vi "Delete.vi"(0 "video in":refnum<class "MSC Video.lvclass">, 5 "error in (no error)":errorcluster) -> (19 "error out":errorcluster)   [LabVIEW 2014, in "MSC Video.lvclass"]
doc: "Closes the video reference and frees occupied memory.\nUse this function for each initialized video to prevent memory leaks."
uses:
  MSC Video.lvclass
  MSC Video.lvclass/MSC Video.ctl
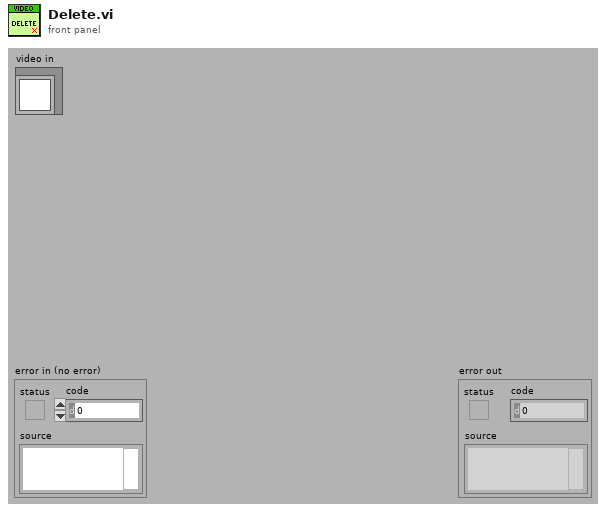
[diagram p1: front panel]
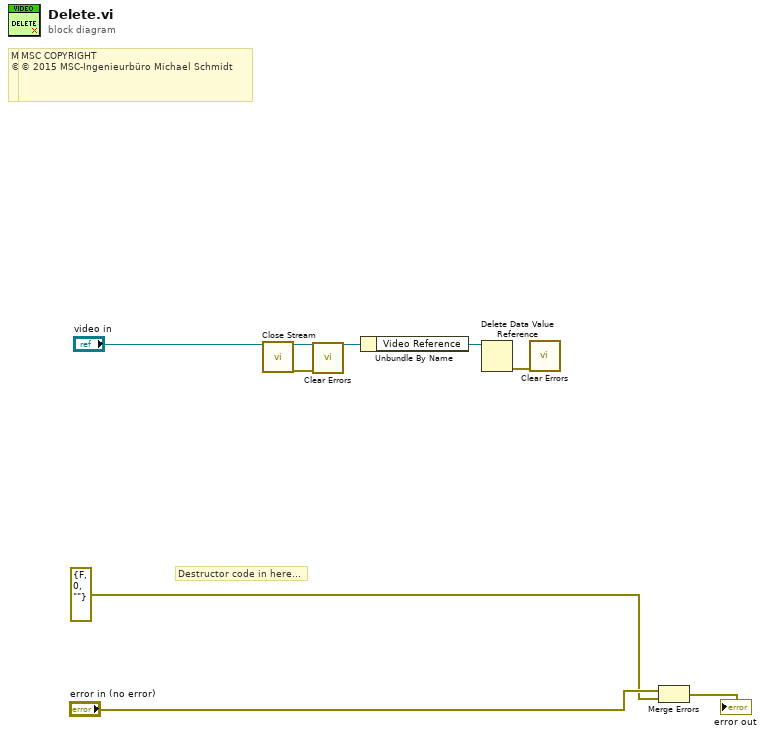
[diagram p0: block diagram]
diagram:
  # "MSC COPYRIGHT\n© 2016 MSC-Ingenieurbüro Michael Schmidt"
  # "MSC COPYRIGHT\n© 2016 MSC-Ingenieurbüro Michael Schmidt"
  # "MSC COPYRIGHT\n© 2015 MSC-Ingenieurbüro Michael Schmidt"
  # "Destructor code in here..."
  n1 = call-dynamic "Close Stream.vi"("video in"="video in") -> ("video out"=w1:refnum<class "MSC Video.lvclass">, "error out"=w5:errorcluster)  [unwired: 17 in]
  n2 = call <vilib>:"Clear Errors.vi"("error in (no error)"=w5) -> ()  [unwired: 5 in, 2 out]
  n3 = Unbundle By Name(w1) -> ("Video Reference"=w4:refnum<data-value>)
  n4 = Delete Data Value Reference(data value reference=w4) -> (error out=w3:errorcluster)  [unwired: 1 in, 1 out]
  n5 = call <vilib>:"Clear Errors.vi"("error in (no error)"=w3) -> ()  [unwired: 5 in, 2 out]
  n6 = Merge Errors("error in (no error)", errorcluster {"status"=FALSE, "code"=0, "source"=""} ("error in (no error)")) -> (→"error out":errorcluster)
